vi "test_PinMapWrapper_StopPinMapService_WrapperMethodsWorkWithoutError.vi"(8 "error in":errorcluster) -> (0 "error out":errorcluster, 2 "result":string, 3 "pass":bool)   [LabVIEW 2020, in "MeasurementServerTests.lvlib" / "TestStand Integration Tests.lvlib"]
uses:
  TestStand Integration Tests.lvlib
  Helpers/Pin Map XML Strings Global.vi
  MeasurementServerTests.lvlib
  Runtime/MeasurementLink TestStand Integration/MeasurementLink TestStand Integration.lvlib
  Runtime/MeasurementLink Pin Map Client/RPC Messages/ni_measurementlink_pinmap_v1_UpdatePinMapFromXmlRequest.ctl
  Runtime/MeasurementLink Pin Map Client/MeasurementLink Pin Map Client.lvlib
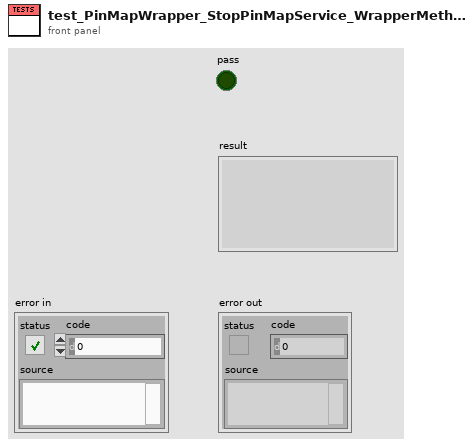
[diagram p1: front panel]
types:
  T1 = typedef "MeasurementLink Pin Map Client.lvlib/ni_measurementlink_pinmap_v1_UpdatePinMapFromXmlRequest.ctl" = cluster{"pin_map_id":string, "pin_map_xml":string}
  T2 = typedef "MeasurementLink Pin Map Client.lvlib/ni_measurementlink_pinmap_v1_PinMap.ctl" = cluster{"pin_map_id":string}
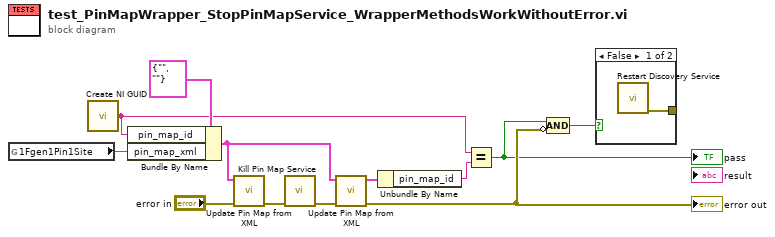
[diagram p0: block diagram]
diagram:
  n1 = global read "Pin Map XML Strings Global.vi" "1Fgen1Pin1Site"() -> (w8:string)
  n2 = call <vilib>:"Create NI GUID.vi"() -> ("NI GUID"=w7:string)
  n3 = Bundle By Name(cluster=T1 {"pin_map_id"="", "pin_map_xml"=""} ("request data"), "pin_map_id"=w7, "pin_map_xml"=w8) -> (w1:T1)
  n4 = call "Update Pin Map from XML.vi"("error in"="error in", "request data"=w1) -> ("error out"=w2:errorcluster)  [unwired: 8 in, 1 out]
  n5 = call "Kill Pin Map Service.vi"("error in"=w2) -> ("error out"=w10:errorcluster)  [unwired: 10 in]
  n6 = call "Update Pin Map from XML.vi"("error in"=w10, "request data"=w1) -> ("error out"=w11:errorcluster, "response data"=w6:T2)  [unwired: 8 in]
  "error out" <- w11
  n7 = Unbundle By Name(w6) -> ("pin_map_id"=w5:string)
  n8 = Equal?(x=w7, y=w5) -> (x = y?=w4:bool)
  "pass" <- w4
  n9 = Compound Arithmetic op=AND(w4, invert w11) -> (w12:bool)
  n10 = case shown="False" w12 {
    tunnel: [w13 _] -> _
    frame False {
      n11 = call "Restart Discovery Service.vi"() -> ("error out"=w13:errorcluster)  [unwired: 11 in]
    }
    frame True {
    }
  }
